vi "Field Draw Balls.vi"(4 "Draw Targets?":T1, 6 "balls":T2[](array[typedef]), 8 "Picture In":picture, 9 "Offset":cluster{"Width":dbl, "Height":dbl}, 10 "Scale":dbl, 11 "Balls":T3[](array[typedef])) -> (0 "Picture Out":picture, 1 "Offset Out":cluster{"Width":dbl, "Height":dbl}, 2 "Scale Out":dbl)   [LabVIEW 2016]
uses:
  SSL Detection Ball.ctl
  <vilib>/Analysis/Matrix/Datatypes/RealMatrix.ctl
  Core/AI Ball.ctl
  DrawTargets.ctl
  <vilib>/Analysis/Matrix/NI_Matrix.lvlib
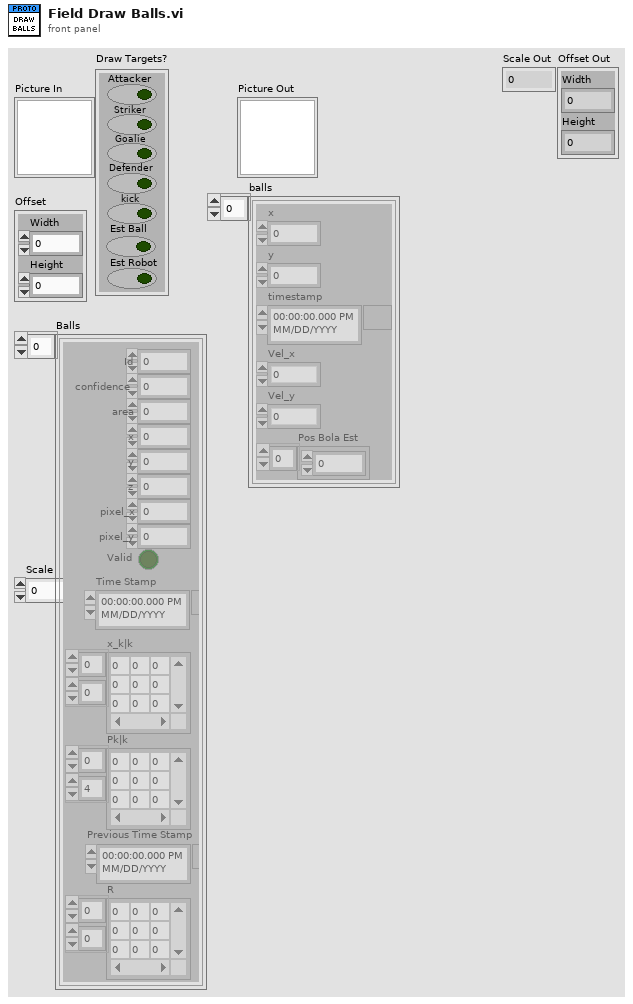
[diagram p1: front panel]
types:
  T1 = typedef "DrawTargets.ctl" = cluster{"Attacker":bool, "Striker":bool, "Goalie":bool, "Defender":bool, "kick":bool, "Est Ball":bool, "Est Robot":bool}
  T2 = typedef "AI Ball.ctl" = cluster{"x":dbl, "y":dbl, "timestamp":timestamp, "Vel_x":dbl, "Vel_y":dbl, "Pos Bola Est":dbl[]}
  T3 = typedef "SSL Detection Ball.ctl" = cluster{"x":sgl, "area":u32, "confidence":sgl, "y":sgl, "z":sgl, "pixel_x":sgl, "pixel_y":sgl, "Valid":bool, "Time Stamp":timestamp, "x_k|k":T4, "Pk|k":T4, "Id":u32, "Previous Time Stamp":timestamp, "R":T4}
  T4 = typedef "NI_Matrix.lvlib/RealMatrix.ctl" = dbl[][]
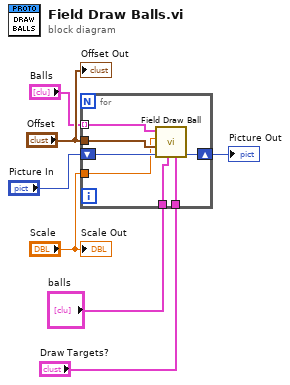
[diagram p0: block diagram]
diagram:
  n1 = for {
    tunnel: "Scale" -> [w10]
    tunnel: "Offset" -> [w11]
    tunnel: "Balls" -> [w12] mode=indexing
    shift-right: [w14] -> w4
    shift-left: "Picture In" -> [w13]
    tunnel: "balls" -> [w9]
    tunnel: "Draw Targets?" -> [w8]
    n2 = call "Field Draw Ball.vi"("Draw Targets?"=w8, "balls"=w9, "picture in"=w13, "Offset"=w11, "Scale mm/pixel"=w10, "Detection Ball"=w12) -> ("picture out"=w14:picture)  [unwired: 5 in]
  }
  "Picture Out" <- w4
  "Scale Out" <- "Scale"
  "Offset Out" <- "Offset"
